vi "Update.vi"(8 "Error In":errorcluster, 11 "I/O Control":T1) -> (0 "Error Out":errorcluster)   [LabVIEW 2019, in "sbRIO9623.lvlib"]
uses:
  SubVI/IO Control.ctl
  sbRIO9623.lvlib
  Queues/Queues.lvlib
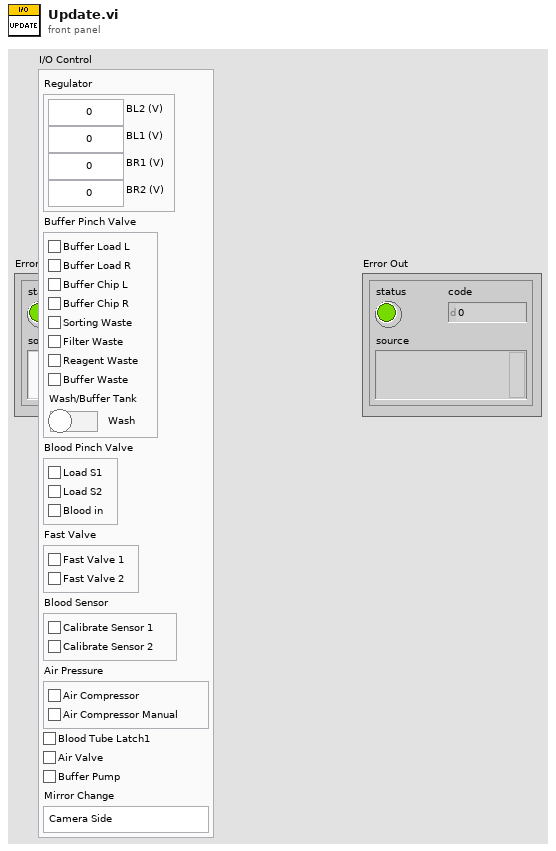
[diagram p1: front panel]
types:
  T1 = typedef "sbRIO9623.lvlib/IO Control.ctl" = cluster{"Regulator":cluster{"BL2 (V)":fxp<+,16,3>, "BL1 (V)":fxp<+,16,3>, "BR1 (V)":fxp<+,16,3>, "BR2 (V)":fxp<+,16,3>}, "Buffer Pinch Valve":cluster{"Buffer Load L":bool, "Buffer Load R":bool, "Buffer Chip L":bool, "Buffer Chip R":bool, "Sorting Waste":bool, "Filter Waste":bool, "Reagent Waste":bool, "Buffer Waste":bool, "Wash/Buffer Tank":bool}, "Blood Pinch Valve":cluster{"Load S1":bool, "Load S2":bool, "Blood in":bool}, "Fast Valve":cluster{"Fast Valve 1":bool, "Fast Valve 2":bool}, "Blood Sensor":cluster{"Calibrate Sensor 1":bool, "Calibrate Sensor 2":bool}, "Air Pressure":cluster{"Air Compressor":bool, "Air Compressor Manual":bool}, "Blood Tube Latch1":bool, "Air Valve":bool, "Buffer Pump":bool, "Mirror Change":enum16{"Camera Side", "SiPM Side"}}
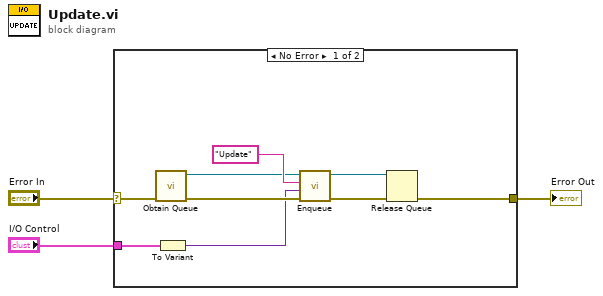
[diagram p0: block diagram]
diagram:
  n1 = case shown="No Error" "Error In" {
    selector: "Error In" -> [w8 w13]
    tunnel: [w9 w13] -> w3
    tunnel: "I/O Control" -> [w5 _]
    frame No Error {
      n2 = call "Obtain Queue.vi"("Error In"=w8) -> ("Error Out"=w7:errorcluster, "Queue out"=w6:refnum<queue>)  [unwired: 9 in]
      n3 = To Variant(anything=w5) -> (Variant=w4:variant)
      n4 = call "Enqueue.vi"("Error In"=w7, "Data"=w4, "State"="Update", "Queue in"=w6) -> ("Error Out"=w11:errorcluster, "Queue out"=w10:refnum<queue>)  [unwired: 6 in]
      n5 = Release Queue(queue=w10, error in (no error)=w11) -> (error out=w9:errorcluster)  [unwired: 1 in, 2 out]
    }
    frame Error {
    }
  }
  "Error Out" <- w3
